vi "test con 492.vi"(4 "Numeric":i32, 5 "Puerto:":u16, 7 "IP":string) -> (0 "Text.Text Colors:Text Color":u32, 1 "Text.Text Colors:Text Color 2":u32, 2 "TEST? 2":string, 3 "TEST?":string, 6 "error out":errorcluster)   [LabVIEW 2010]
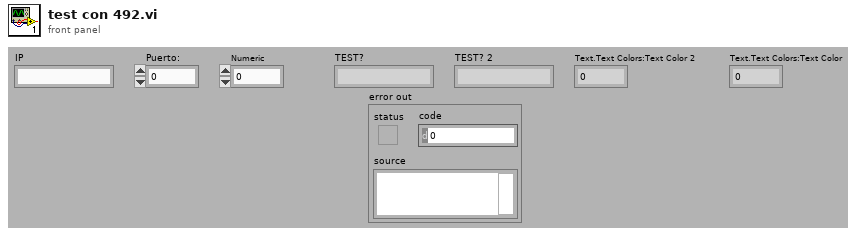
[diagram p1: front panel]
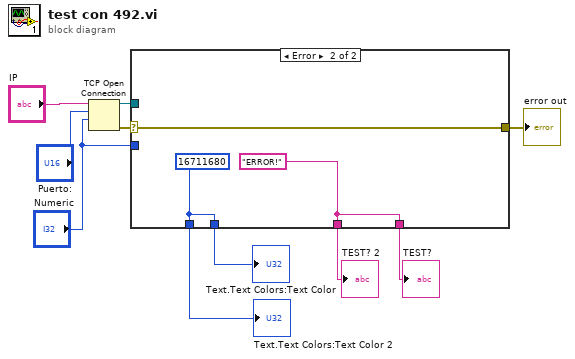
[diagram p0: block diagram]
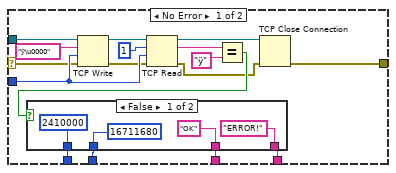
[diagram p2: hidden frame]
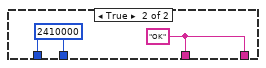
[diagram p3: hidden frame]
diagram:
  n1 = TCP Open Connection(address="IP", remote port or service name="Puerto:", timeout ms (60000)="Numeric") -> (connection ID=w4:refnum<k5>, error out=w9:errorcluster)  [unwired: 1 in, 1 out]
  n2 = case shown="Error" w9 {
    selector: w9 -> [w12 w34]
    tunnel: w4 -> [w27 _]
    tunnel: [w17 w35] -> w7
    tunnel: [w22 w36] -> w5
    tunnel: "Numeric" -> [w24 _]
    tunnel: [w19 w36] -> w6
    tunnel: [w18 w35] -> w8
    tunnel: [w11 w34] -> w1
    frame No Error {
      n3 = TCP Write(connection ID=w27, data in="ÿ\u0000", error in (no error)=w12, 9:w24) -> (connection ID out=w25:refnum<k5>, error out=w14:errorcluster)  [unwired: 1 out]
      n4 = TCP Read(connection ID=w25, bytes to read=1, error in (no error)=w14, 9:w24) -> (connection ID out=w21:refnum<k5>, data out=w16:string, error out=w13:errorcluster)  [unwired: 1 out]
      n5 = Equal?(x=w16, y="ÿ" ("data in")) -> (x = y?=w20:bool)
      n6 = case shown="False" w20 {
        tunnel: ["OK" ("TEST?") w33] -> w17
        tunnel: [u32 2410000 ("Text.Text Colors\n:Text Color") w32] -> w22
        tunnel: [u32 16711680 ("Text.Text Colors:Text Color") w32] -> w19
        tunnel: ["ERROR!" ("TEST?") w33] -> w18
        frame False {
        }
        frame True {
          w33 = "OK" ("TEST?")
          w32 = u32 2410000 ("Text.Text Colors\n:Text Color")
        }
      }
      n7 = TCP Close Connection(connection ID=w21, error in (no error)=w13) -> (error out=w11:errorcluster)  [unwired: 2 out]
    }
    frame Error {
      w36 = u32 16711680 ("Text.Text Colors:Text Color")
      w35 = "ERROR!" ("TEST?")
    }
  }
  "TEST?" <- w8
  "TEST? 2" <- w7
  "Text.Text Colors:Text Color" <- w6
  "Text.Text Colors:Text Color 2" <- w5
  "error out" <- w1
